vi "String To Variant.vi"(10 "Type":T1 {"Number" items=["? One or none"=0, "* Any"=-1, "+ At least one"=-2]}, 11 "String":string) -> (0 "error out":errorcluster, 3 "Variant":variant)   [LabVIEW 2020, in "LV ArgParse.lvlib" / "LV Argument Parser.lvclass"]
uses:
  LV Argument Parser.lvclass
  <vilib>/Utility/error.llb/Error Cluster From Error Code.vi
  <vilib>/ErrorRing/Error Ring.xnode
  Argument Definition.ctl
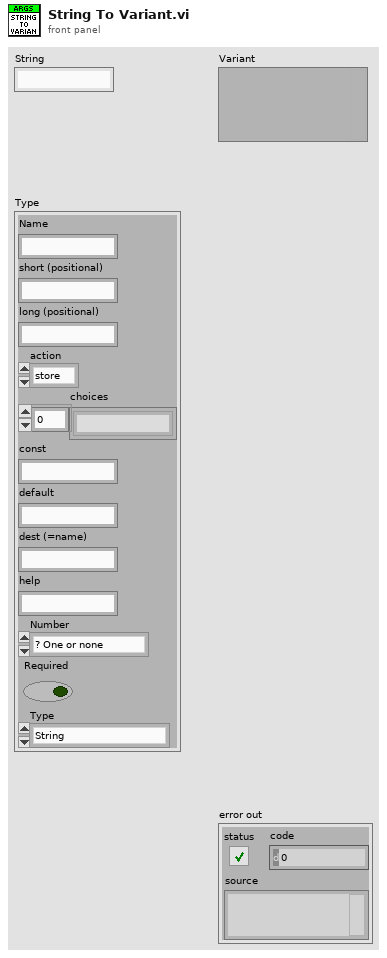
[diagram p1: front panel]
types:
  T1 = typedef "LV ArgParse.lvlib/LV Argument Parser.lvclass/Argument Definition.ctl" = cluster{"Name":string, "short (positional)":string, "long (positional)":string, "action":enum16{"store", "store-const", "store-false", "store-true", "append", "append-const", "count", "help", "version"}, "choices":string[], "const":string, "default":string, "dest (=name)":string, "help":string, "Number":i32, "Required":bool, "Type":enum16{"String", "Int", "UInt", "Float", "Bool", "Date", "Path"}}
  T2 = enum16{"String", "Int", "UInt", "Float", "Bool", "Date", "Path"}
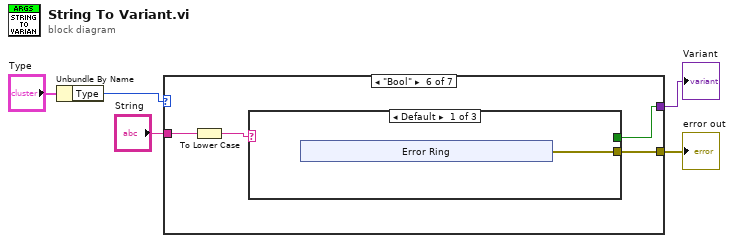
[diagram p0: block diagram]
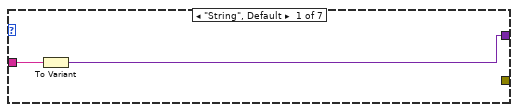
[diagram p2: hidden frame]
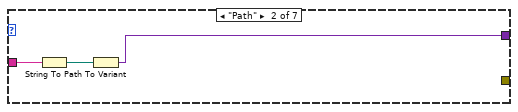
[diagram p3: hidden frame]
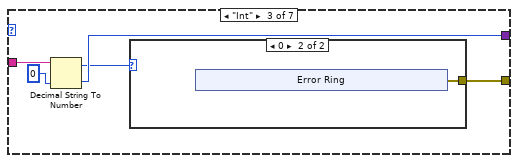
[diagram p4: hidden frame]
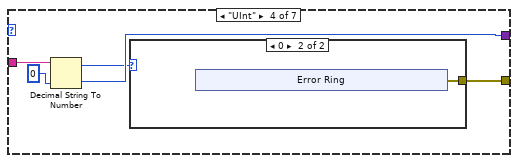
[diagram p6: hidden frame]
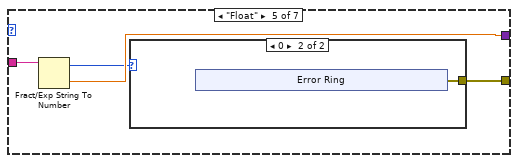
[diagram p8: hidden frame]
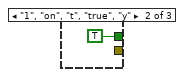
[diagram p10: hidden frame]
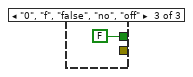
[diagram p11: hidden frame]
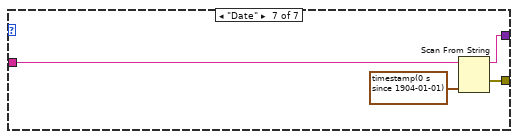
[diagram p12: hidden frame]
diagram:
  n1 = Unbundle By Name("Type") -> ("Type"=w1:T2)
  n2 = case shown="\"Bool\"" w1 {
    tunnel: "String" -> [w7 w10 w15 w25 w34 w43 w53]
    tunnel: [w6 w9 w13 w23 w33 w41 w52] -> w4
    tunnel: [_ _ w12 w21 w32 w40 w51] -> w5
    frame "String", Default {
      n3 = To Variant(anything=w7) -> (Variant=w6:variant)
    }
    frame "Path" {
      n4 = String To Path(string=w10) -> (path=w8:path)
      n5 = To Variant(anything=w8) -> (Variant=w9:variant)
    }
    frame "Int" {
      n6 = Decimal String To Number(string=w15, default (0L)=0 ("default (0 I32)")) -> (offset past number=w11:i32, number=w13:i32)  [unwired: 1 in]
      n7 = case shown="0" w11 {
        tunnel: [_ w16] -> w12
        frame Default {
        }
        frame 0 {
          n8 = xnode "Error Ring"() -> ("error out"=w16:errorcluster)
        }
      }
    }
    frame "UInt" {
      n9 = Decimal String To Number(string=w25, default (0L)=u32 0 ("default (0 I32)")) -> (offset past number=w22:i32, number=w23:u32)  [unwired: 1 in]
      n10 = case shown="0" w22 {
        tunnel: [_ w26] -> w21
        frame Default {
        }
        frame 0 {
          n11 = xnode "Error Ring"() -> ("error out"=w26:errorcluster)
        }
      }
    }
    frame "Float" {
      n12 = Fract/Exp String To Number(string=w34) -> (offset past number=w31:i32, number=w33:dbl)  [unwired: 3 in]
      n13 = case shown="0" w31 {
        tunnel: [_ w35] -> w32
        frame Default {
        }
        frame 0 {
          n14 = xnode "Error Ring"() -> ("error out"=w35:errorcluster)
        }
      }
    }
    frame "Bool" {
      n15 = To Lower Case(string=w43) -> (all lower case string=w42:string)
      n16 = case shown="Default" w42 {
        tunnel: [_ TRUE FALSE] -> w41
        tunnel: [w44 _ _] -> w40
        frame Default {
          n17 = xnode "Error Ring"() -> ("error out"=w44:errorcluster)
        }
        frame "1", "on", "t", "true", "y" {
        }
        frame "0", "f", "false", "no", "off" {
        }
      }
    }
    frame "Date" {
      n18 = Scan From String(input string=w53, default 1=timestamp(0 s since 1904-01-01)) -> (remaining string=w52:string, error out=w51:errorcluster)  [unwired: 4 in, 1 out]
    }
  }
  "error out" <- w5
  "Variant" <- w4
